vi "Utility_RW Cluster Data to File.vi"(7 "System":string="4296 Data", 8 "Error":errorcluster, 9 "Read(f)Write(t)":bool, 10 "Data Name":string="VisonSettings", 11 "Cluster Data":variant) -> (0 "Error Out":errorcluster, 2 "Found? Out":bool, 3 "Cluster Data Out":variant)   [LabVIEW 2017]
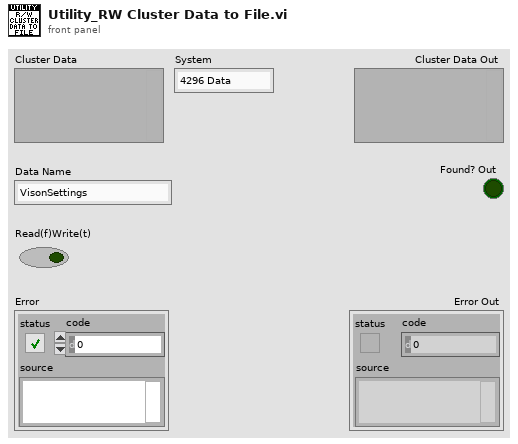
[diagram p1: front panel]
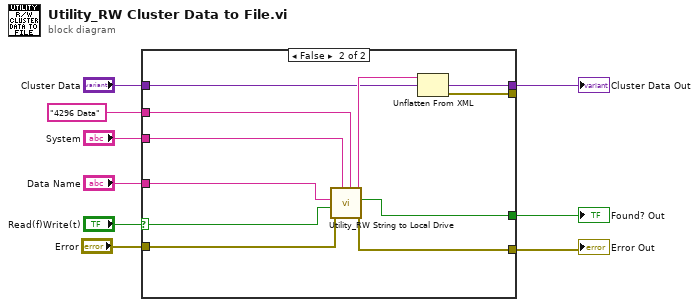
[diagram p0: block diagram]
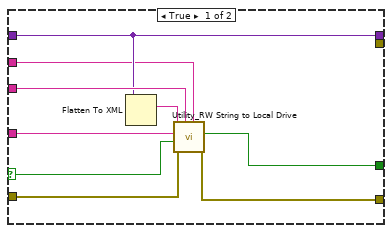
[diagram p2: hidden frame]
diagram:
  n1 = case shown="False" "Read(f)Write(t)" {
    selector: "Read(f)Write(t)" -> [w12 w21]
    tunnel: "Data Name" -> [w18 w29]
    tunnel: "System" -> [w17 w28]
    tunnel: [w16 w27] -> w7
    tunnel: [w15 w26] -> w6
    tunnel: "Error" -> [w14 w25]
    tunnel: [w11 w23] -> w4
    tunnel: "Cluster Data" -> [w11 w22]
    tunnel: [_ w20] -> _
    tunnel: "4296 Data" ("File Name") -> [w10 w19]
    frame True {
      n2 = Flatten To XML(anything=w11) -> (xml string=w13:string)
      n3 = call "Utility_RW String to Local Drive.vi"("File Name"=w10, "System"=w17, "Error"=w14, "Read(f)Write(t)"=w12, "Data Name"=w18, "String Data"=w13) -> ("Error Out"=w15:errorcluster, "Found? Out"=w16:bool)  [unwired: 3 in, 1 out]
    }
    frame False {
      n4 = call "Utility_RW String to Local Drive.vi"("File Name"=w19, "System"=w28, "Error"=w25, "Read(f)Write(t)"=w21, "Data Name"=w29) -> ("Error Out"=w26:errorcluster, "Found? Out"=w27:bool, "String Data Out"=w24:string)  [unwired: 4 in]
      n5 = Unflatten From XML(xml string=w24, type=w22) -> (value=w23:variant, error out=w20:errorcluster)  [unwired: 1 in]
    }
  }
  "Cluster Data Out" <- w4
  "Found? Out" <- w7
  "Error Out" <- w6
